vi "LecturaDatosMotorLabView.vi"() -> ()   [LabVIEW 2025]
uses:
  <vilib>/Utility/file.llb/Write Delimited Spreadsheet (DBL).vi
panel:
  out "Waveform Chart":dynamicdata(graph)
  out "Numeric":dbl
  in  "stop":bool
  in  "Slide":dbl(slide) scale=0.0..5.0
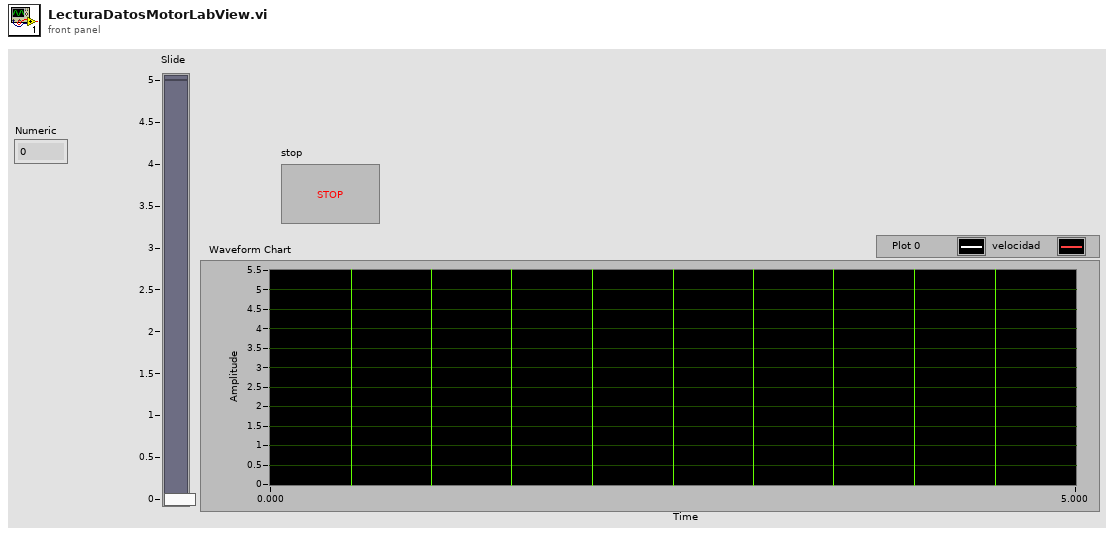
[diagram p1: front panel]
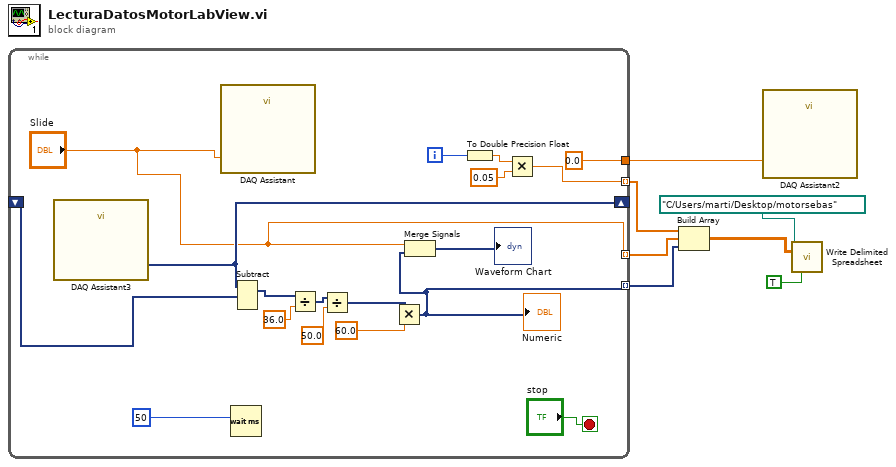
[diagram p0: block diagram]
diagram:
  n1 = while {
    tunnel: [0.0 ("Numeric")] -> w7
    shift-right: [w15] -> _
    shift-left: _ -> [w14]
    tunnel: ["Slide"] -> w3 mode=indexing
    tunnel: [w12] -> w4 mode=indexing
    tunnel: [w9] -> w6 mode=indexing
    i -> [w10]
    stop <- "stop" stop-if-true
    n2 = call "DAQ Assistant3"() -> ("data"=w15:dynamicdata)  [unwired: 16 in, 3 out]
    n3 = call "DAQ Assistant"("data"="Slide") -> ()  [unwired: 17 in, 2 out]
    n4 = Wait (ms)(milliseconds to wait=u32 50 ("millisecond timer value")) -> ()  [unwired: 1 out]
    n5 = Subtract(1:w14, 2:w15) -> (0:w22:dynamicdata)  [unwired: 1 in, 1 out]
    n6 = Divide(x=w22, y=36.0 ("Numeric")) -> (x/y=w23:dynamicdata)
    n7 = Divide(x=w23, y=50.0 ("Numeric")) -> (x/y=w19:dynamicdata)
    n8 = Multiply(x=w19, y=60.0 ("Numeric")) -> (x*y=w12:dynamicdata)
    "Numeric" <- w12
    n9 = Merge Signals("Slide", w12) -> (→"Waveform Chart":dynamicdata)
    n10 = To Double Precision Float(number=w10) -> (double precision float=w11:dbl)
    n11 = Multiply(x=w11, y=0.05) -> (x*y=w9:dbl)
  }
  n12 = Build Array(w6, w3, w4) -> (w1:dbl[][])
  n13 = call "DAQ Assistant2"("data"=w7) -> ()  [unwired: 17 in, 2 out]
  n14 = call-poly <vilib>:"Write Delimited Spreadsheet.vi"("file path (dialog if empty)"=path "C:/Users/marti/Desktop/motorsebas", "2D data"=w1, "transpose? (no:F)"=TRUE) -> ()  [unwired: 11 in, 2 out]
